vi "Init.vi"(8 "error in (no error)":errorcluster, 11 "Effect Interface in":refnum<class "Effect Interface.lvclass">) -> (0 "error out":errorcluster, 3 "Effect Interface out":refnum<class "Effect Interface.lvclass">)   [LabVIEW 2019, in "Effect Interface.lvlib" / "Effect Interface.lvclass"]
uses:
  Effect Interface.lvclass
  Effect Interface.lvclass/Effect Interface.ctl
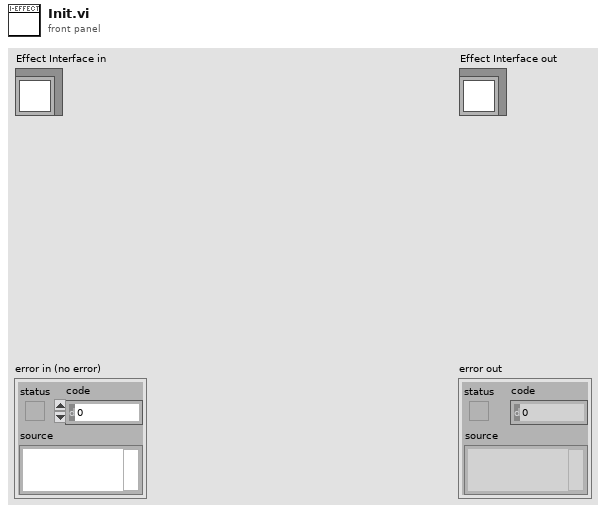
[diagram p1: front panel]
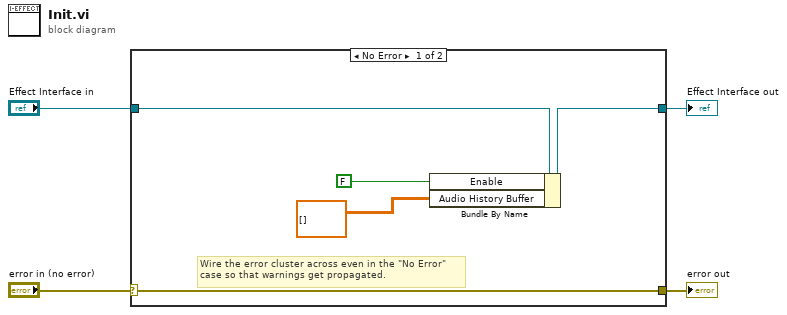
[diagram p0: block diagram]
diagram:
  n1 = case shown="No Error" "error in (no error)" {
    selector: "error in (no error)" -> [w9 w11]
    tunnel: [w9 w11] -> w3
    tunnel: [w5 w10] -> w1
    tunnel: "Effect Interface in" -> [w6 w10]
    frame No Error {
      # "Wire the error cluster across even in the \"No Error\"\ncase so that warnings get propagated."
      n2 = Bundle By Name(cluster=w6, "Enable"=FALSE, "Audio History Buffer"=dbl[][] []) -> (w5:refnum<class "Effect Interface.lvclass">)
    }
    frame Error {
    }
  }
  "error out" <- w3
  "Effect Interface out" <- w1
